vi "Notfi_Creat.vi"(8 "error in (no error)":errorcluster, 11 "NotifyIcon in":refnum<class "NotifyIcon.lvclass">) -> (0 "error out":errorcluster, 3 "NotifyIcon out":refnum<class "NotifyIcon.lvclass">)   [LabVIEW 2016, in "NotifyIcon.lvclass"]
uses:
  NotifyIcon.lvclass
  System.Windows.Forms
  NotifyIcon.lvclass/NotifyIcon.ctl
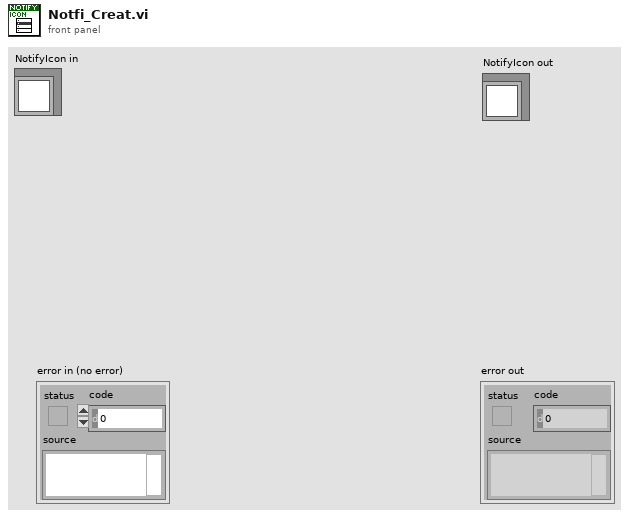
[diagram p1: front panel]
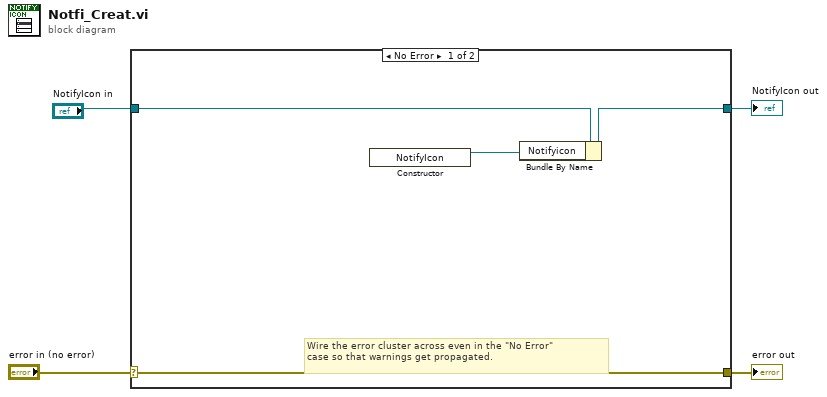
[diagram p0: block diagram]
diagram:
  n1 = case shown="No Error" "error in (no error)" {
    selector: "error in (no error)" -> [w8 w10]
    tunnel: [w8 w10] -> w3
    tunnel: [w6 w9] -> w1
    tunnel: "NotifyIcon in" -> [w7 w9]
    frame No Error {
      # "Wire the error cluster across even in the \"No Error\"\ncase so that warnings get propagated."
      n2 = constructor class="NotifyIcon"() -> (reference out=w5:refnum<k24>)  [unwired: 3 in, 2 out]
      n3 = Bundle By Name(cluster=w7, "Notifyicon"=w5) -> (w6:refnum<class "NotifyIcon.lvclass">)
    }
    frame Error {
    }
  }
  "error out" <- w3
  "NotifyIcon out" <- w1
